vi "Command_tool.vi"() -> ()   [LabVIEW 2018]
panel:
  out "Triggers":u32[](graph)
  out "timetags":u32[][](array[numeric])
  out "detections":u32[](graph)
  in  "Number of repetitions":i32
  in  "repetitions":i32
  in  "q_samples":i32=100
  in  "stop_us":dbl=300.0 min=0.01
  in  "start_us":dbl=0.01 min=0.01
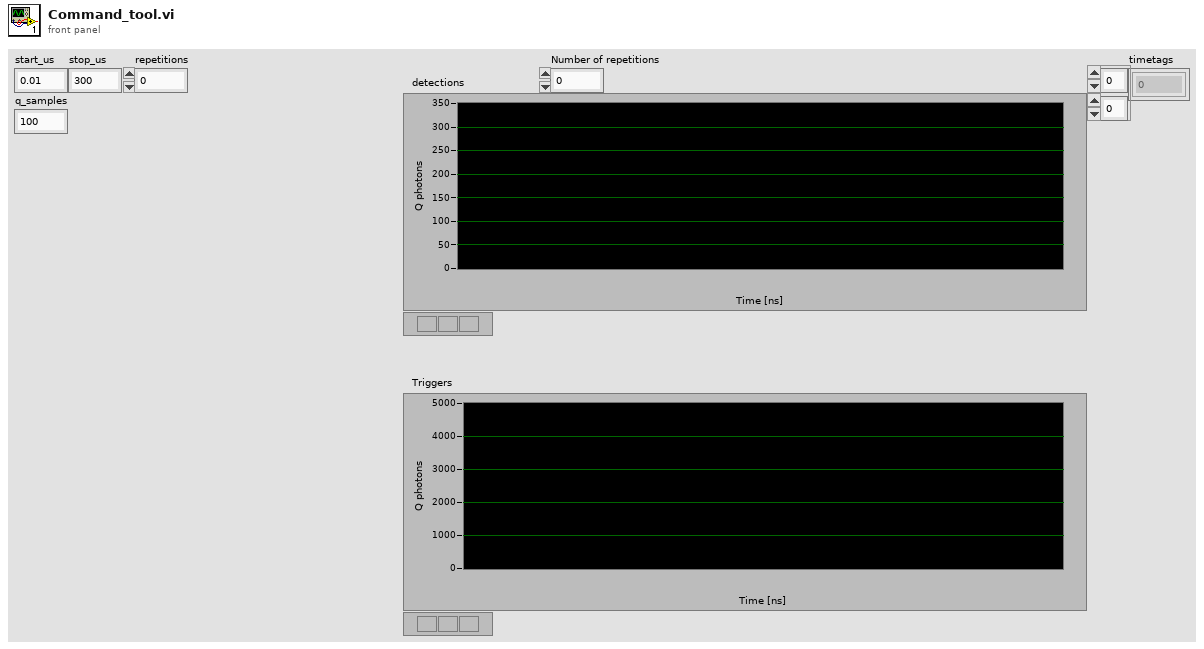
[diagram p1: front panel]
types:
  T1 = cluster{"dark_times_us":dbl[], "pulse_width_us":dbl, "read_delay_us":dbl, "read_width_us":dbl, "repetitions":i32, "sampling_mode":enum16{"Normal", "Sweep"}, "correction_us":dbl}
  T2 = cluster{"MW_width_us":dbl[], "pulse_width_us":dbl, "read_delay_us":dbl, "read_width_us":dbl, "repetitions":i32, "sampling_mode":enum16{"Normal", "Sweep"}, "correction_us":dbl}
  T3 = cluster{"Instruct Data":i32, "Op Code":i32, "Flags":bool[], "Comments":string, "Time":dbl}[]
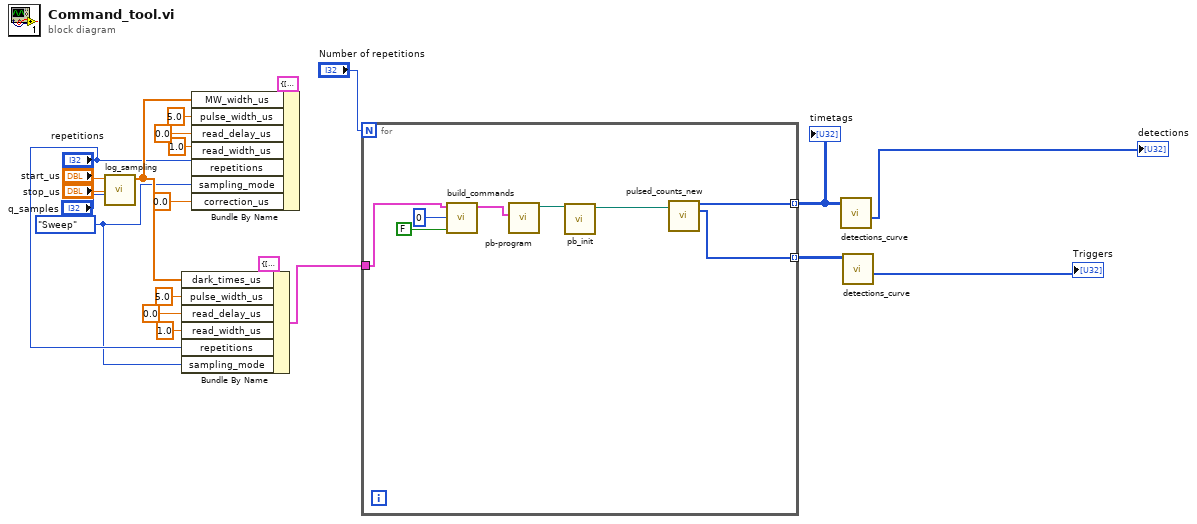
[diagram p0: block diagram]
diagram:
  w2 = enum16{"Normal", "Sweep"}."Sweep" ("sampling_mode")
  n1 = call "log_sampling.vi"("q_samples"="q_samples", "stop_us"="stop_us", "start_us"="start_us") -> ("sampling_times_us"=w7:dbl[])  [unwired: 7 in, 1 out]
  n2 = Bundle By Name(cluster=T1 {"dark_times_us"=[1.0, 31.624000000000002, 1000.0], "pulse_width_us"=5.0, "read_delay_us"=0.0, "read_width_us"=1.0, "repetitions"=100000, "sampling_mode"=enum."Sweep", "correction_us"=0.65} ("T1_parameters"), "dark_times_us"=w7, "pulse_width_us"=5.0, "read_delay_us"=0.0, "read_width_us"=1.0, "repetitions"="repetitions", "sampling_mode"=w2) -> (w1:T1)
  n3 = Bundle By Name(cluster=T2 {"MW_width_us"=[], "pulse_width_us"=0.0, "read_delay_us"=0.0, "read_width_us"=0.0, "repetitions"=0, "sampling_mode"=enum."Normal", "correction_us"=0.0} ("Rabi_parameters"), "MW_width_us"=w7, "pulse_width_us"=5.0, "read_delay_us"=0.0, "read_width_us"=1.0, "repetitions"="repetitions", "sampling_mode"=w2, "correction_us"=0.0) -> ()  [unwired: 1 out]
  n4 = for {
    N: "Number of repetitions" -> [_]
    tunnel: [w27] -> w12 mode=indexing
    tunnel: [w26] -> w10 mode=indexing
    tunnel: w1 -> [w25]
    n5 = call "build_commands.vi"("Refocus_s"=u32 0, "Refocus?"=FALSE, "T1_parameters"=w25) -> ("instructions_array"=w24:T3)  [unwired: 8 in]
    n6 = call "pb-program.vi"("Commands"=w24) -> ("path out"=w23:path)  [unwired: 10 in]
    n7 = call "pb_init.vi"("path in"=w23) -> ("path out"=w22:path)  [unwired: 9 in, 1 out]
    n8 = call "pulsed_counts_new.vi"("path in"=w22) -> ("timetags"=w27:u32[], "triggers"=w26:u32[])  [unwired: 10 in, 3 out]
  }
  "timetags" <- w12
  n9 = call "detections_curve.vi"("timetags"=w12) -> ("detections"=→"detections":u32[])  [unwired: 10 in]
  n10 = call "detections_curve.vi"("timetags"=w10) -> ("detections"=→"Triggers":u32[])  [unwired: 10 in]
